vi "Read_Value_From_Excel.vi"(0 "Excel._Application":refnum<k7>, 1 "Excel File Path":path=path "C:/Documents and Settings/rquintal/Desktop/TestParameters.xls", 7 "Row":string="1", 9 "Column":string="a", 11 "error in (no error)":errorcluster, 12 "Worksheet":string="Sheet1", 13 "Open new instance(T)":bool=TRUE, 14 "Close application (T)":bool=TRUE) -> (4 "Excel._Application Out":refnum<k7>, 6 "Data from Cell":string="key", 15 "error out":errorcluster)   [LabVIEW 2018]
doc: "This example program demonstrates how to read a value from a particular cell in an Excel spreadsheet. Specify the path to an excel file, the worksheet number, and the cell to read and run the VI. The data in the specified file will appear on the front panel."
panel:
  in  "Row 2":string="1"
  in  "Column 2":string="a"
  # "Select Help»Show Context Help and move the cursor over the VI icon to display help for this VI"
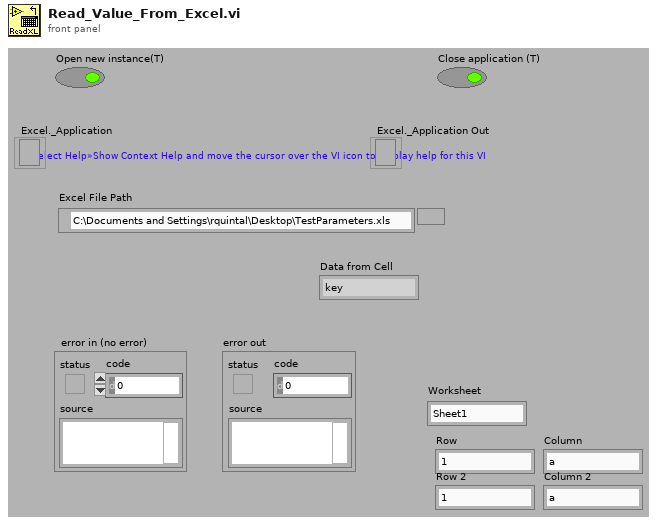
[diagram p1: front panel]
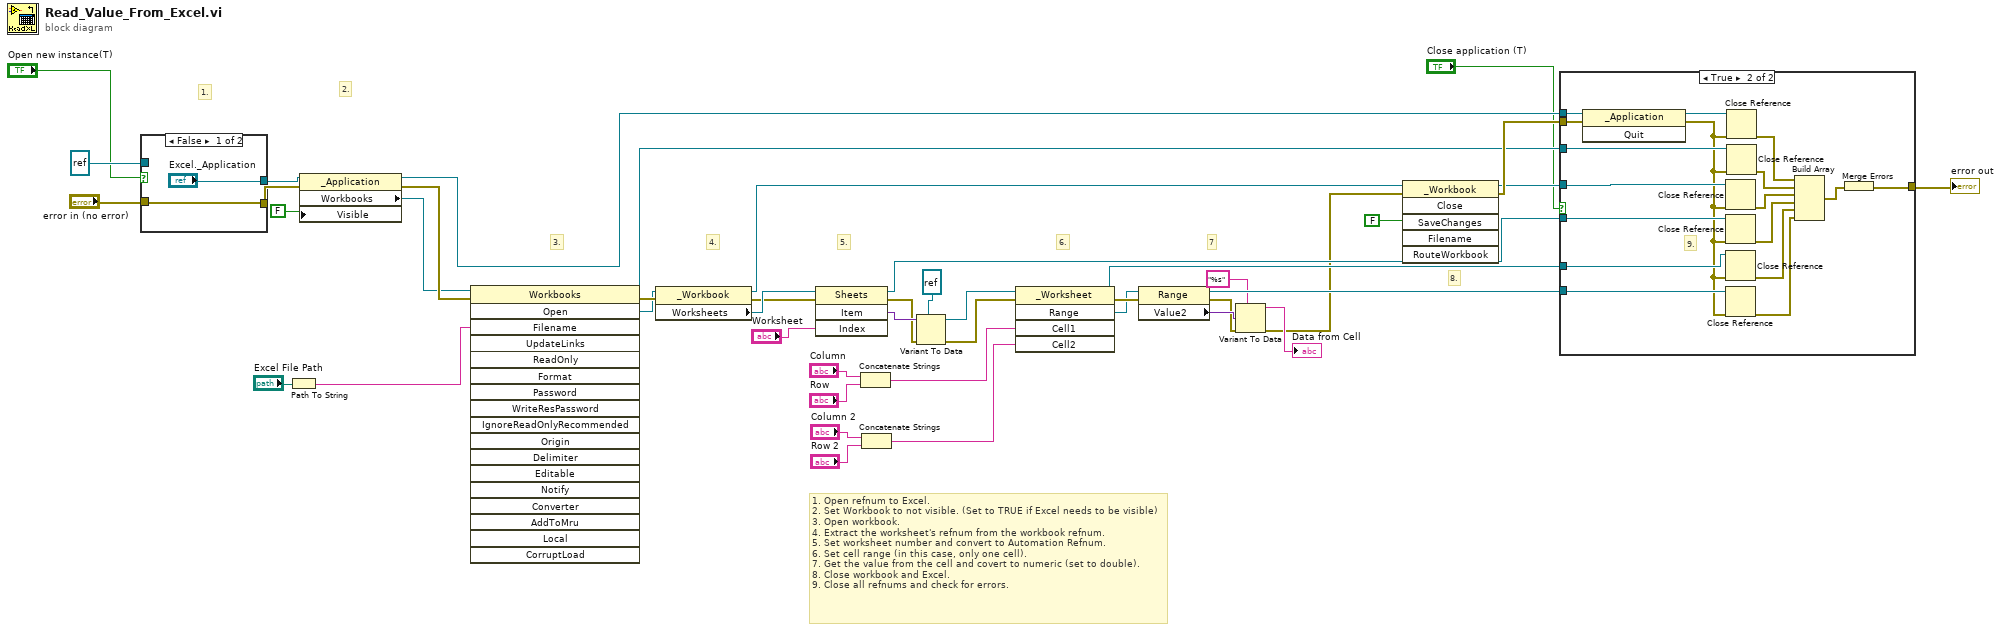
[diagram p0: block diagram]
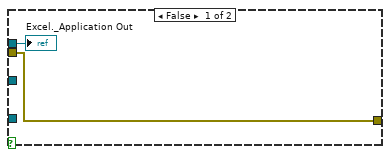
[diagram p2: hidden frame]
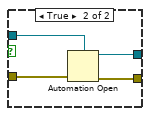
[diagram p3: hidden frame]
diagram:
  # "1. Open refnum to Excel.\n2. Set Workbook to not visible. (Set to TRUE if Excel needs to be visible)\n3. Open workbook.\n4. Extract the worksheet's refnum from the workbook refnum.\n5. Set worksheet number and convert to Automation Refnum.\n6. Set cell range (in this case, only one cell).\n7. Get the value from the cell and covert to numeric (set to double).\n8. Close workbook and Excel.\n9. Close all refnums and check for errors."
  # "8."
  # "7"
  # "6."
  # "5."
  # "4."
  # "3."
  # "2."
  # "1."
  n1 = case shown="False" "Open new instance(T)" {
    tunnel: refnum<k7> refnum ("Excel._Application") -> [_ w50]
    tunnel: "error in (no error)" -> [w45 w49]
    tunnel: ["Excel._Application" w48] -> w42
    tunnel: [w45 w47] -> w41
    frame False {
    }
    frame True {
      n2 = Automation Open(error in (no error)=w49, Automation Refnum=w50) -> (Automation Refnum=w48:refnum<k7>, error out=w47:errorcluster)  [unwired: 2 in]
    }
  }
  n3 = Path To String(path="Excel File Path") -> (string=w36:string)
  n4 = property class="_Application"(reference=w42, error in=w41, "Visible"=FALSE) -> (reference out=w16:refnum<k7>, error out=w39:errorcluster, "Workbooks"=w38:refnum<k7>)
  n5 = invoke class="Workbooks" method="Open"(reference=w38, error in=w39, "Filename"=w36) -> (reference out=w7:refnum<k7>, error out=w35:errorcluster, "Open"=w34:refnum<k7>)  [unwired: 15 in, 15 out]
  n6 = property class="_Workbook"(reference=w34, error in=w35) -> (reference out=w19:refnum<k7>, error out=w32:errorcluster, "Worksheets"=w33:refnum<k7>)
  n7 = invoke class="Sheets" method="Item"(reference=w33, error in=w32, "Index"="Worksheet") -> (reference out=w23:refnum<k7>, error out=w29:errorcluster, "Item"=w30:variant)  [unwired: 1 in, 1 out]
  n8 = Concatenate Strings("Column", "Row") -> (w9:string)
  n9 = Concatenate Strings("Column 2", "Row 2") -> (w2:string)
  n10 = Variant To Data(error in=w29, type=refnum<k7> refnum ("Excel._Worksheet"), Variant=w30) -> (data=w28:refnum<k7>, error out=w27:errorcluster)
  n11 = invoke class="_Worksheet" method="Range"(reference=w28, error in=w27, "Cell1"=w9, "Cell2"=w2) -> (reference out=w22:refnum<k7>, error out=w26:errorcluster, "Range"=w12:refnum<k7>)  [unwired: 1 in, 2 out]
  n12 = property class="Range"(reference=w12, error in=w26) -> (reference out=w21:refnum<k7>, error out=w8:errorcluster, "Value2"=w25:variant)
  n13 = Variant To Data(error in=w8, type="%s", Variant=w25) -> (data=→"Data from Cell":string, error out=w17:errorcluster)
  n14 = invoke class="_Workbook" method="Close"(reference=w19, error in=w17, "SaveChanges"=FALSE) -> (reference out=w14:refnum<k7>, error out=w15:errorcluster)  [unwired: 3 in, 4 out]
  n15 = case shown="True" "Close application (T)" {
    tunnel: w23 -> [_ w69]
    tunnel: w22 -> [_ w68]
    tunnel: w21 -> [_ w67]
    tunnel: [w51 w66] -> w20
    tunnel: w16 -> [w52 w65]
    tunnel: w15 -> [w51 w64]
    tunnel: w14 -> [_ w63]
    tunnel: w7 -> [_ w62]
    frame False {
      "Excel._Application Out" <- w52
    }
    frame True {
      # "9."
      n16 = invoke class="_Application" method="Quit"(reference=w65, error in=w64) -> (reference out=w53:refnum<k7>, error out=w54:errorcluster)  [unwired: 1 in, 1 out]
      n17 = Close Reference(reference=w63, error in (no error)=w54) -> (error out=w59:errorcluster)
      n18 = Close Reference(reference=w69, error in (no error)=w54) -> (error out=w58:errorcluster)
      n19 = Close Reference(reference=w68, error in (no error)=w54) -> (error out=w57:errorcluster)
      n20 = Close Reference(reference=w67, error in (no error)=w54) -> (error out=w56:errorcluster)
      n21 = Close Reference(reference=w53, error in (no error)=w54) -> (error out=w61:errorcluster)
      n22 = Close Reference(reference=w62, error in (no error)=w54) -> (error out=w60:errorcluster)
      n23 = Build Array(w61, w60, w59, w58, w57, w56) -> (w55:errorcluster[])
      n24 = Merge Errors(w55) -> (w66:errorcluster)
    }
  }
  "error out" <- w20
